vi "子VI.vi"(5 "ID":string, 7 "Value":refnum<user-event>, 8 "Stop":refnum<user-event>, 9 "Show":refnum<user-event>, 11 "Panel":refnum<class "Panel.lvclass">) -> ()   [LabVIEW 2016]
uses:
  <vilib>/MGI/Panel Manager/Panel/Panel/Panel.lvclass
panel:
  in  "停止发送":bool
  in  "开始发送":bool
  out "波形图表":dbl(graph)
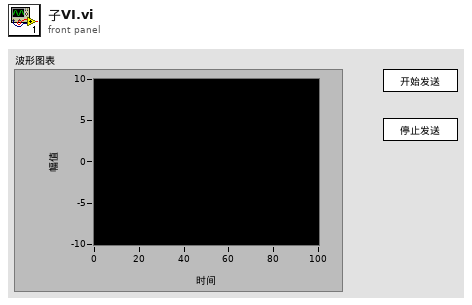
[diagram p1: front panel]
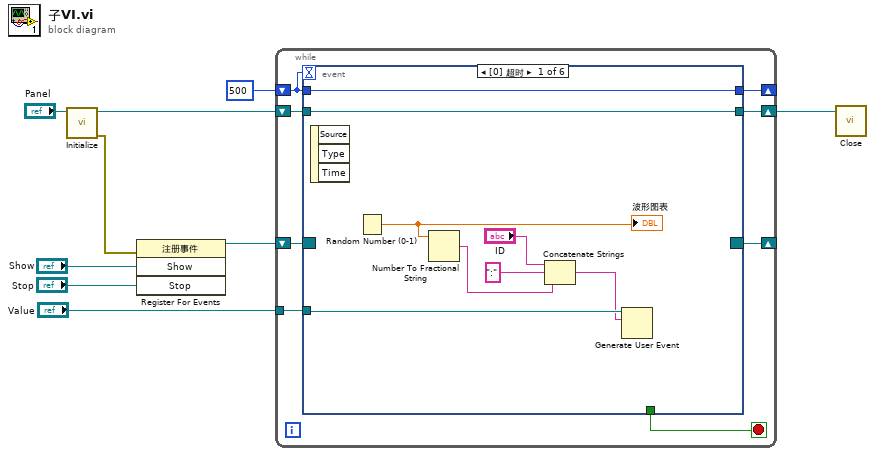
[diagram p0: block diagram]
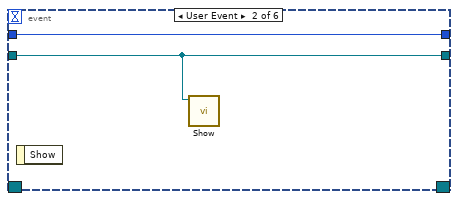
[diagram p2: hidden frame]
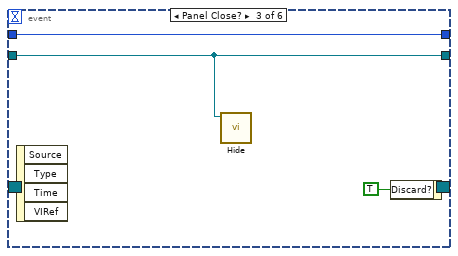
[diagram p3: hidden frame]
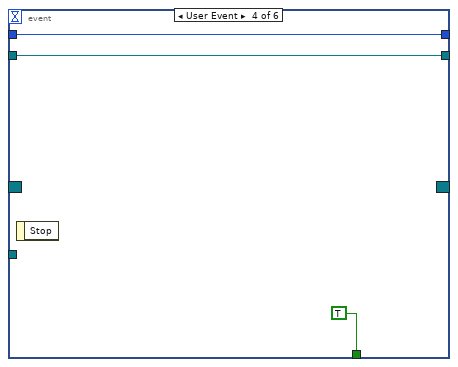
[diagram p4: hidden frame]
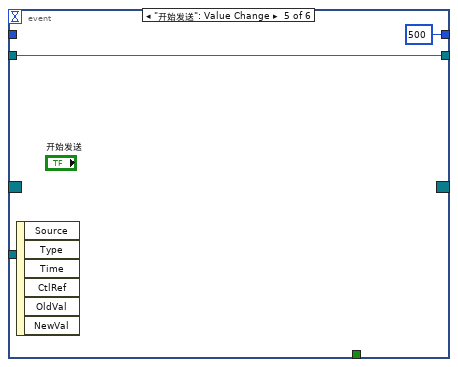
[diagram p5: hidden frame]
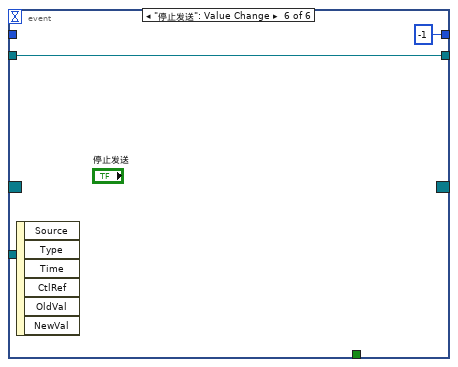
[diagram p6: hidden frame]
diagram:
  n1 = call <vilib>:"Initialize.vi"("Panel In"="Panel") -> ("error out"=w4:errorcluster, "Panel Out"=w8:refnum<class "Panel.lvclass">)  [unwired: 8 in, 1 out]
  n2 = register-events(error in=w4, "Show", "Stop") -> (reference out=w7:refnum<event-registration>)  [unwired: 1 in, 1 out]
  n3 = while {
    shift-right: [w16] -> w3
    shift-left: w8 -> [w17]
    shift-right: [w14] -> _
    shift-left: w7 -> [w15]
    shift-right: [w11] -> _
    shift-left: 500 -> [w12]
    tunnel: "Value" -> [w10]
    stop <- w13 stop-if-true
    n4 = event shown="[0] 超时" {
      selector: w15 -> [_ _ _ _ _ _]
      dyn-events: [_ _ _ _ _ _] -> w14
      timeout: w12 -> [_ _ _ _ _ _]
      tunnel: w17 -> [w25 w27 w29 w33 w34 w36]
      tunnel: [w25 w27 w29 w33 w34 w36] -> w16
      tunnel: [_ _ _ TRUE _ _] -> w13
      tunnel: w12 -> [w18 w26 w28 w31 _ _]
      tunnel: [w18 w26 w28 w31 500 -1] -> w11
      tunnel: w10 -> [w23 _ _ _ _ _]
      event Timeout {
        n5 = event-data() -> ()  [unwired: 1 in, 3 out]
        n6 = Random Number (0-1)() -> (number: 0 to 1=w24:dbl)
        "波形图表" <- w24
        n7 = Number To Fractional String(number=w24) -> (F-format string=w20:string)  [unwired: 3 in]
        n8 = Concatenate Strings("ID", ":" ("字符串"), w20) -> (w19:string)
        n9 = Generate User Event(user event=w23, event data cluster=w19) -> ()  [unwired: 2 in, 2 out]
      }
      event User Event {
        n10 = event-data() -> ()  [unwired: 1 in, 1 out]
        n11 = call <vilib>:"Show.vi"("Panel in"=w27) -> ()  [unwired: 10 in, 1 out]
      }
      event Panel Close? {
        n12 = event-data() -> ()  [unwired: 1 in, 4 out]
        n13 = call <vilib>:"Hide.vi"("Panel In"=w29) -> ()  [unwired: 10 in, 1 out]
        n14 = event-data("Discard?"=TRUE) -> ()  [unwired: 1 in, 1 out]
      }
      event User Event {
        n15 = event-data() -> ()  [unwired: 1 in, 1 out]
      }
      event "开始发送": Value Change {
        n16 = event-data() -> ()  [unwired: 1 in, 6 out]
      }
      event "停止发送": Value Change {
        n17 = event-data() -> ()  [unwired: 1 in, 6 out]
      }
    }
  }
  n18 = call-dynamic "Close.vi"("Panel In"=w3) -> ()  [unwired: 10 in, 1 out]
